vi "SUB_UUT_DatTime_convert.vi"(3 "UUT_DateTime_input":string="20140703155955") -> (1 "UUT TimeStamp out":timestamp)   [LabVIEW 2011]
panel:
  out "UUT sec":i32
  out "UUT min":i32
  out "UUT hour":i32
  out "UUT Day":i32
  out "UUT  Month":i32
  out "UUT Year":i32
  out "size(s)":i32
  out "unsigned byte array":u8[](array[numeric])
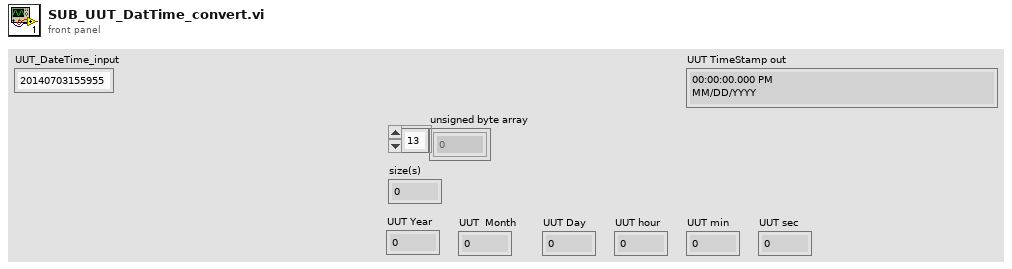
[diagram p1: front panel]
types:
  T1 = cluster{dbl, i32, i32, i32, i32, i32, i32, i32, i32, i32}
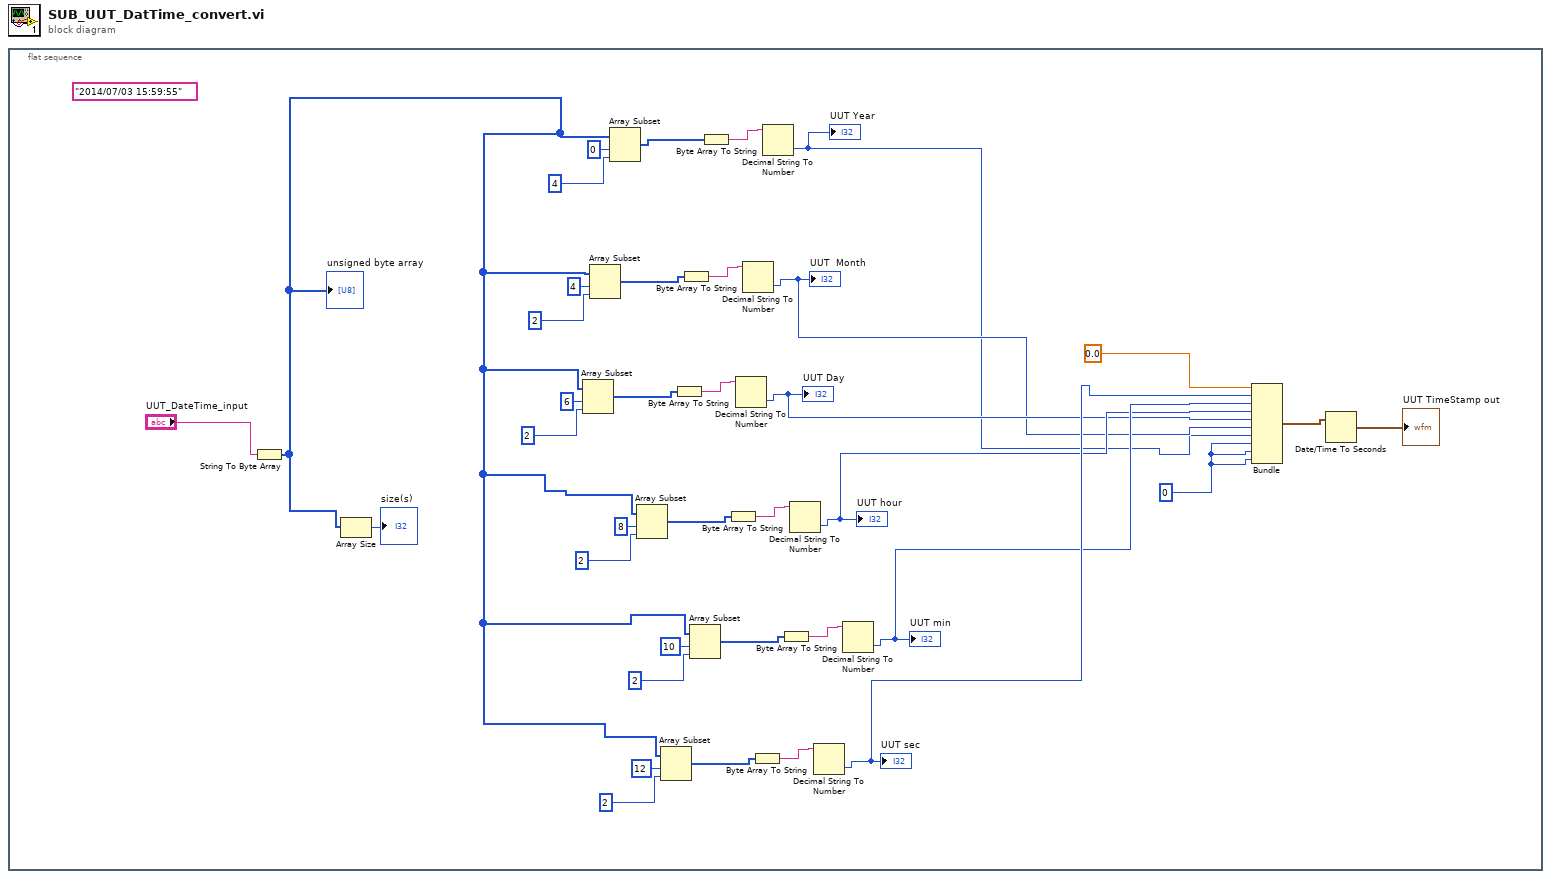
[diagram p0: block diagram]
diagram:
  n1 = flat-sequence {
    frame #0 {
      w3 = 0
      (unwired) "2014/07/03 15:59:55"
      n2 = String To Byte Array(string="UUT_DateTime_input") -> (unsigned byte array=w11:u8[])
      "unsigned byte array" <- w11
      n3 = Array Size(array=w11) -> (size(s)=→"size(s)":i32)
      n4 = Array Subset(array=w11, index=6, length=2 ("index")) -> (w24:u8[])
      n5 = Array Subset(array=w11, index=4, length=2 ("index")) -> (w28:u8[])
      n6 = Array Subset(array=w11, index=0, length=4 ("index")) -> (w35:u8[])
      n7 = Array Subset(array=w11, index=8, length=2 ("index")) -> (w20:u8[])
      n8 = Array Subset(array=w11, index=12, length=2 ("index")) -> (w12:u8[])
      n9 = Byte Array To String(unsigned byte array=w24) -> (string=w25:string)
      n10 = Byte Array To String(unsigned byte array=w28) -> (string=w29:string)
      n11 = Array Subset(array=w11, index=10, length=2 ("index")) -> (w16:u8[])
      n12 = Byte Array To String(unsigned byte array=w35) -> (string=w32:string)
      n13 = Byte Array To String(unsigned byte array=w20) -> (string=w21:string)
      n14 = Decimal String To Number(string=w25) -> (number=w6:i32)  [unwired: 2 in, 1 out]
      "UUT Day" <- w6
      n15 = Decimal String To Number(string=w29) -> (number=w5:i32)  [unwired: 2 in, 1 out]
      "UUT  Month" <- w5
      n16 = Byte Array To String(unsigned byte array=w12) -> (string=w13:string)
      n17 = Decimal String To Number(string=w32) -> (number=w4:i32)  [unwired: 2 in, 1 out]
      "UUT Year" <- w4
      n18 = Byte Array To String(unsigned byte array=w16) -> (string=w17:string)
      n19 = Decimal String To Number(string=w21) -> (number=w7:i32)  [unwired: 2 in, 1 out]
      "UUT hour" <- w7
      n20 = Decimal String To Number(string=w13) -> (number=w9:i32)  [unwired: 2 in, 1 out]
      "UUT sec" <- w9
      n21 = Decimal String To Number(string=w17) -> (number=w8:i32)  [unwired: 2 in, 1 out]
      "UUT min" <- w8
      n22 = Bundle(0.0, w9, w8, w7, w6, w5, w4, w3, w3, w3) -> (w2:T1)  [unwired: 1 in]
      n23 = Date/Time To Seconds(2:w2) -> (0:→"UUT TimeStamp out":timestamp)  [unwired: 1 in]
    }
  }
